vi "SetWindowAlwaysOnTop.vi"(8 "No Error":errorcluster, 10 "On Top":bool, 11 "Window [SDL_Window *]":T1 format="%.0x") -> (0 "Error Out":errorcluster)   [LabVIEW 2026, in "SDL3.lvlib" / "Video.lvlib"]
doc: "<B>Summary</B>\nSet the window to always be above the others.\n\n<B>Remarks</B>\nThis will add or remove the window's <B>SDL_WINDOW_ALWAYS_ON_TOP</B> flag. This will bring the window to the front and keep the window above the rest."
uses:
  Video.lvlib
  <vilib>/Utility/error.llb/Error Cluster From Error Code.vi
  Error/Error.lvlib
  Lib/SDL3.dll
  SDL_Window--pointer.ctl
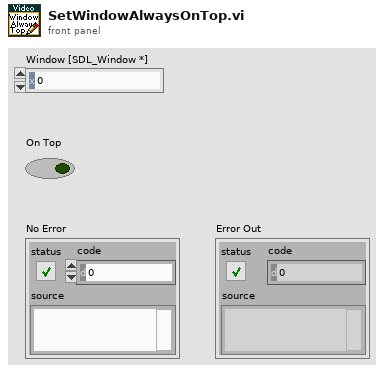
[diagram p1: front panel]
types:
  T1 = typedef "SDL3.lvlib/Video.lvlib/SDL_Window--pointer.ctl" = i64
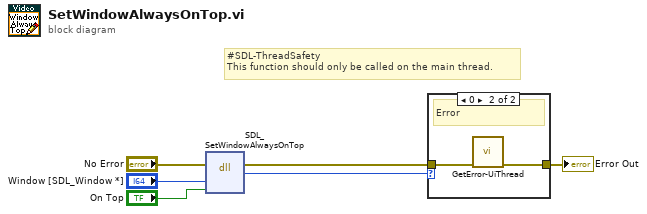
[diagram p0: block diagram]
diagram:
  # "#SDL-ThreadSafety\nThis function should only be called on the main thread."
  n1 = dll-call lib="C:/Users/saukko/Dev/LV-SDL3/Sources/SDL3/Lib/SDL3.*" fn="SDL_SetWindowAlwaysOnTop"(error in="No Error", "window"="Window [SDL_Window *]", "on_top"="On Top") -> (error out=w3:errorcluster, "return type"=w2:i32)  [unwired: 4 in, 1 out]
  n2 = case shown="0" w2 {
    tunnel: w3 -> [w7 w9]
    tunnel: [w7 w8] -> w5
    frame Default {
      # "Ok"
    }
    frame 0 {
      # "Error"
      n3 = call "GetError-UiThread.vi"("No Error"=w9) -> ("error out"=w8:errorcluster)  [unwired: 10 in]
    }
  }
  "Error Out" <- w5
